vi "_script_fix_exclude event case ref check.vi"   [LabVIEW 2014]
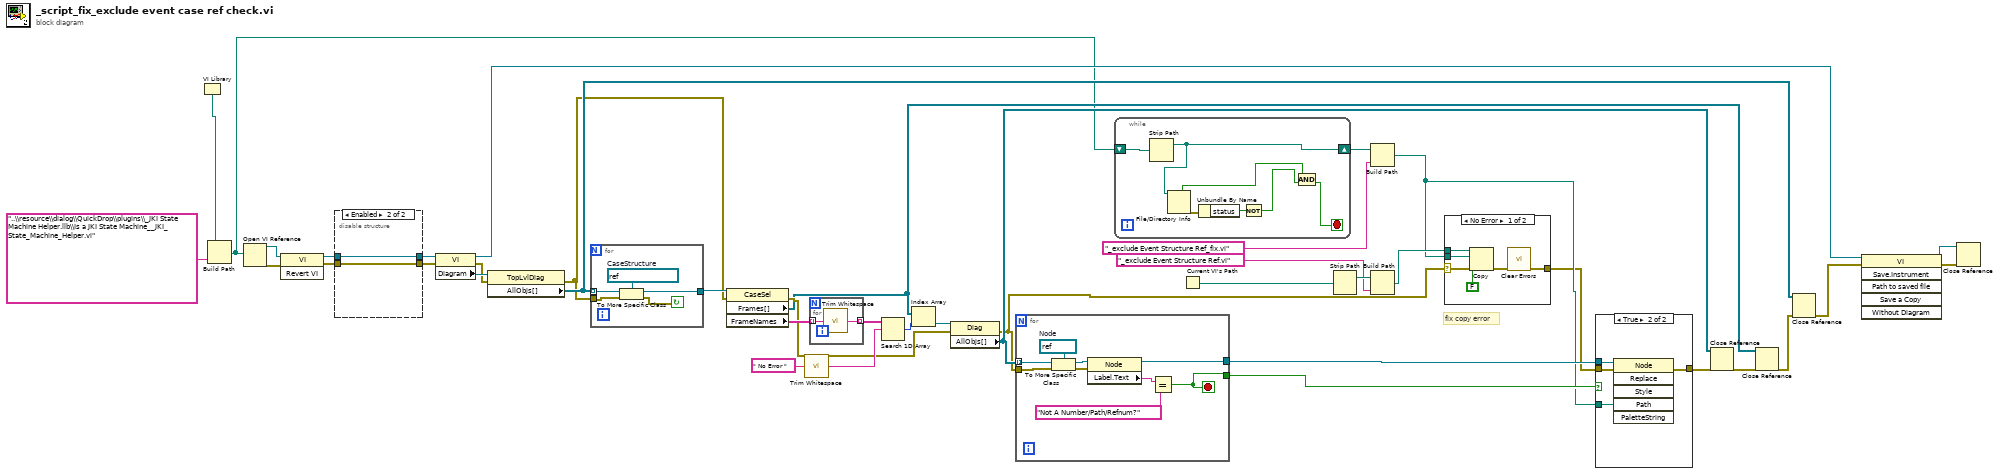
[diagram p0: block diagram]
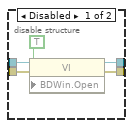
[diagram p3: hidden frame]
diagram:
  # "fix copy error"
  n1 = VI Library() -> (path=w39:path)
  n2 = Build Path(base path=w39, name or relative path="..\\resource\\dialog\\QuickDrop\\plugins\\_JKI State Machine Helper.llb\\Is a JKI State Machine__JKI_State_Machine_Helper.vi") -> (appended path=w7:path)
  n3 = Open VI Reference(vi path=w7) -> (vi reference=w40:refnum<vi>, error out=w41:errorcluster)  [unwired: 5 in]
  n4 = invoke class="VI" method="Revert VI"(reference=w40, error in=w41) -> (reference out=w35:refnum<vi>, error out=w34:errorcluster)  [unwired: 1 in, 1 out]
  n5 = disable-structure shown="Enabled" {
    disable-tunnel: w35 -> [w46 w48]
    disable-tunnel: w34 -> [w45 w47]
    disable-tunnel: [w44 w48] -> w33
    disable-tunnel: [w43 w47] -> w32
    frame Disabled {
      n6 = property class="VI"(reference=w46, error in=w45, "BDWin.Open"=TRUE ("Block Diagram Window:Open")) -> (reference out=w44:refnum<vi>, error out=w43:errorcluster)
    }
    frame Enabled {
    }
  }
  n7 = property class="VI"(reference=w33, error in=w32) -> (reference out=w28:refnum<vi>, error out=w30:errorcluster, "Diagram"=w31:refnum<vi>)
  n8 = property class="TopLvlDiag"(reference=w31, error in=w30) -> (error out=w19:errorcluster, "AllObjs[]"=w26:refnum<vi>[])  [unwired: 1 out]
  n9 = for {
    tunnel: w26 -> [w53] mode=indexing
    tunnel: [w49] -> w29
    tunnel: w19 -> [w51]
    stop <- w50 continue-if-true
    w52 = refnum<vi> refnum  # CaseStructure
    n10 = To More Specific Class(target class=w52, reference=w53, error in=w51) -> (specific class reference=w49:refnum<vi>, error out=w50:errorcluster)
  }
  n11 = property class="CaseSel"(reference=w29, error in=w19) -> (error out=w18:errorcluster, "Frames[]"=w12:refnum<vi>[], "FrameNames"=w25:string[])  [unwired: 1 out]
  n12 = call <vilib>:"Trim Whitespace.vi"("string"=" No Error " ("element")) -> ("trimmed string"=w22:string)  [unwired: 1 in]
  n13 = for {
    tunnel: w25 -> [w55] mode=indexing
    tunnel: [w54] -> w23 mode=indexing
    n14 = call <vilib>:"Trim Whitespace.vi"("string"=w55) -> ("trimmed string"=w54:string)  [unwired: 1 in]
  }
  n15 = Search 1D Array(1D array=w23, element=w22) -> (index of element=w21:i32)  [unwired: 1 in]
  n16 = Index Array(array=w12, index=w21) -> (element=w20:refnum<vi>)
  n17 = property class="Diag"(reference=w20, error in=w18) -> (error out=w5:errorcluster, "AllObjs[]"=w13:refnum<vi>[])  [unwired: 1 out]
  n18 = for {
    tunnel: w13 -> [w64] mode=indexing
    tunnel: w5 -> [w62]
    tunnel: [w57] -> w17
    tunnel: [w56] -> w4
    stop <- w56 stop-if-true
    w63 = refnum<vi> refnum  # Node
    n19 = To More Specific Class(target class=w63, reference=w64, error in=w62) -> (specific class reference=w61:refnum<vi>, error out=w60:errorcluster)
    n20 = property class="Node"(reference=w61, error in=w60) -> (reference out=w57:refnum<vi>, "Label.Text"=w59:string)  [unwired: 1 out]
    n21 = Equal?(x=w59, y="Not A Number/Path/Refnum?") -> (x = y?=w56:bool)
  }
  n22 = while {
    shift-right: [w67] -> w8
    shift-left: w7 -> [w71]
    stop <- w70 stop-if-true
    n23 = Strip Path(path=w71) -> (stripped path=w67:path)  [unwired: 1 out]
    n24 = File/Directory Info(path=w67) -> (directory=w66:bool, error out=w69:errorcluster)  [unwired: 1 in, 5 out]
    n25 = Unbundle By Name(w69) -> ("status"=w68:bool)
    n26 = Not(x=w68) -> (.not. x?=w65:bool)
    n27 = And(x=w66, y=w65) -> (x .and. y?=w70:bool)
  }
  n28 = Current VI's Path() -> (path=w16:path)
  n29 = Strip Path(path=w16) -> (stripped path=w15:path)  [unwired: 1 out]
  n30 = Build Path(base path=w8, name or relative path="_exclude Event Structure Ref_fix.vi") -> (appended path=w3:path)
  n31 = Build Path(base path=w15, name or relative path="_exclude Event Structure Ref.vi") -> (appended path=w9:path)
  n32 = case shown="No Error" w5 {
    selector: w5 -> [w75 w78]
    tunnel: w9 -> [w77 _]
    tunnel: w3 -> [w73 _]
    tunnel: [w72 w78] -> w1
    frame No Error {
      n33 = Copy(8:w75, 9:FALSE ("overwrite (F)"), 10:w73, 11:w77) -> (0:w74:errorcluster)  [unwired: 1 in, 2 out]
      n34 = call <vilib>:"Clear Errors.vi"("error in (no error)"=w74) -> ("error out"=w72:errorcluster)  [unwired: 6 in]
    }
    frame Error {
    }
  }
  n35 = case shown="True" w4 {
    tunnel: w17 -> [_ w83]
    tunnel: [w79 w82] -> w14
    tunnel: w1 -> [w79 w81]
    tunnel: w3 -> [_ w80]
    frame False {
    }
    frame True {
      n36 = invoke class="Node" method="Replace"(reference=w83, error in=w81, "Path"=w80) -> (error out=w82:errorcluster)  [unwired: 3 in, 5 out]
    }
  }
  n37 = Close Reference(reference=w13, error in (no error)=w14) -> (error out=w11:errorcluster)
  n38 = Close Reference(reference=w12, error in (no error)=w11) -> (error out=w10:errorcluster)
  n39 = Close Reference(reference=w26, error in (no error)=w10) -> (error out=w27:errorcluster)
  n40 = invoke class="VI" method="Save.Instrument"(reference=w28, error in=w27) -> (reference out=w36:refnum<vi>, error out=w37:errorcluster)  [unwired: 4 in, 4 out]
  n41 = Close Reference(reference=w36, error in (no error)=w37) -> ()  [unwired: 1 out]
